vi "Trav_move_above_height.vi"(4 "Currently on Point":i32=11, 6 "Row Number":i32=11, 7 "Extra Command String":string, 8 "Simulate/Run":T1, 9 "Backlash Compensation?":bool=TRUE, 10 "New Position":dbl[](array[numeric])=[0.0, 0.0, 0.0] format="%.2f", 11 "Mode":T2) -> (0 "Error String":string, 3 "Trav Position achieved":dbl[](array[numeric]) format="%.2f")   [LabVIEW 2010]
uses:
  Trav_mode.ctl
  Controls/User_Specific_mode.ctl
  Globals/Trav_pos_global.vi
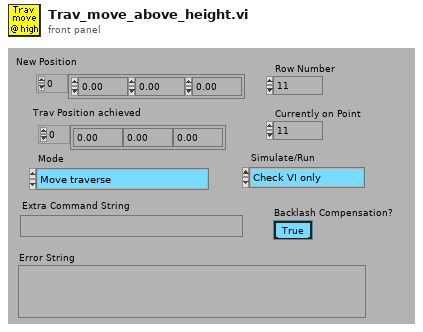
[diagram p1: front panel]
types:
  T1 = typedef "User_Specific_mode.ctl" = enum16{"Check VI only", "Run VI"}
  T2 = typedef "Trav_mode.ctl" = enum16{"Move traverse", "Read traverse position", "Teach Position"}
  T3 = typedef "Tunnel_Coordinates.ctl" = enum16{"Work in Tunnel Coordinates", "Work in Model Coordinates"}
  T4 = enum16{"To Traverse Coordinates", "To User Coordinates"}
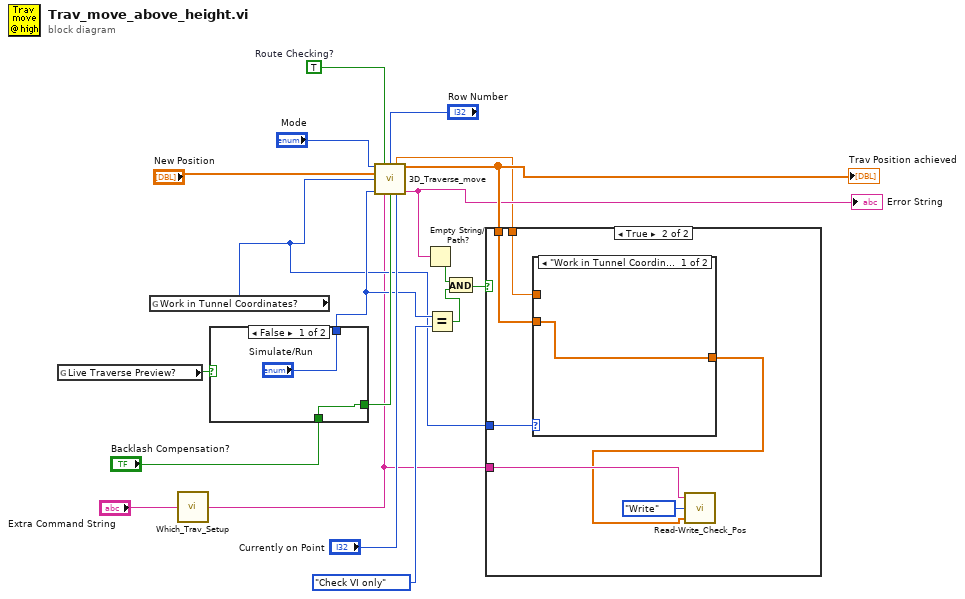
[diagram p0: block diagram]
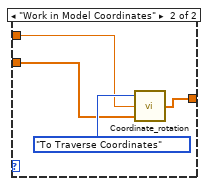
[diagram p3: hidden frame]
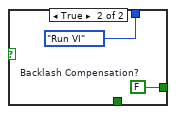
[diagram p4: hidden frame]
diagram:
  w11 = TRUE  # Route Checking?
  n1 = global read "Trav_pos_global.vi" "Live Traverse Preview?"() -> (w13:bool)
  n2 = global read "Trav_pos_global.vi" "Work in Tunnel Coordinates?"() -> (w4:T3)
  n3 = call "Which_Trav_Setup.vi"("Extra Command String"="Extra Command String") -> ("Traverse Setup"=w3:string)
  n4 = case shown="False" w13 {
    tunnel: ["Simulate/Run" User_Specific_mode."Run VI" ("Simulate/Run")] -> w9
    tunnel: [w20 w22] -> w12
    tunnel: "Backlash Compensation?" -> [w20 _]
    frame False {
    }
    frame True {
      w22 = FALSE  # Backlash Compensation?
    }
  }
  n5 = call "3D_Traverse_move.vi"("Mode"="Mode", "Route Checking?"=w11, "Row Number"="Row Number", "Position"="New Position", "Work in Tunnel Coordinates"=w4, "Simulate/Run"=w9, "Traverse name"=w3, "Backlash Compensation?"=w12, "Currently on Point"="Currently on Point") -> ("Model Rotation (deg)"=w5:dbl, "Trav Position achieved"=w18:dbl[], "Error String"=w17:string)  [unwired: 4 out]
  "Trav Position achieved" <- w18
  "Error String" <- w17
  n6 = Empty String/Path?(string/path=w17) -> (empty?=w8:bool)
  n7 = Equal?(x=w9, y=User_Specific_mode."Check VI only" ("Simulate/Run")) -> (x = y?=w7:bool)
  n8 = And(x=w8, y=w7) -> (x .and. y?=w6:bool)
  n9 = case shown="True" w6 {
    tunnel: w5 -> [_ w29]
    tunnel: w18 -> [_ w28]
    tunnel: w4 -> [_ w27]
    tunnel: w3 -> [_ w25]
    frame False {
    }
    frame True {
      n10 = case shown="\"Work in Tunnel Coordinates\"" w27 {
        tunnel: w28 -> [w30 w33]
        tunnel: [w30 w32] -> w24
        tunnel: w29 -> [_ w31]
        frame "Work in Tunnel Coordinates" {
        }
        frame "Work in Model Coordinates" {
          n11 = call "Coordinate_rotation.vi"("Input Position"=w33, "Coordinate rotation (deg)"=w31, "Mode"=T4."To Traverse Coordinates") -> ("Output Position"=w32:dbl[])
        }
      }
      n12 = call "Read-Write_Check_Pos.vi"("Position input"=w24, "Mode"=enum16{"Read", "Write"}."Write", "Traverse Name"=w25) -> ()  [unwired: 1 out]
    }
  }
